vi "update if true.vi"() -> ()   [LabVIEW 2010]
panel:
  in  "s":bool
  out "value":i32
  in  "new value":i32
  in  "old value":i32
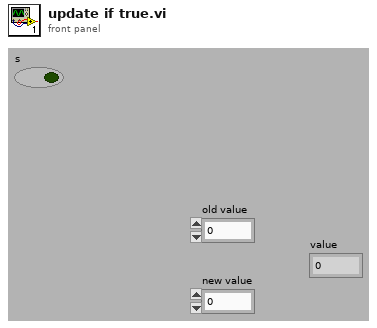
[diagram p1: front panel]
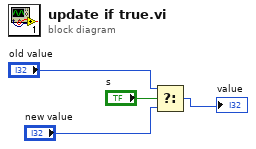
[diagram p0: block diagram]
diagram:
  n1 = Select(t="old value", s="s", f="new value") -> (s? t:f=→"value":i32)
